vi "Read Order Items.vi"(8 "error in (no error)":errorcluster, 11 "Order in":refnum<class "Order.lvclass">) -> (0 "error out":errorcluster, 2 "Items":refnum<class "Order Item.lvclass">[](array[class]), 3 "Order out":refnum<class "Order.lvclass">)   [LabVIEW 2020, in "Order.lvclass"]
doc: "Simple accessor method to read the items contained in the Order."
uses:
  Order.lvclass
  Order Item/Order Item.lvclass
  Order.lvclass/Order.ctl
  Processes/People/Customers/Customer/Customer.lvclass
  C:/Users/anton/Documents/GitHub/Triarc-Examples/Coffee Shop/Process Job/Job Handler.lvclass
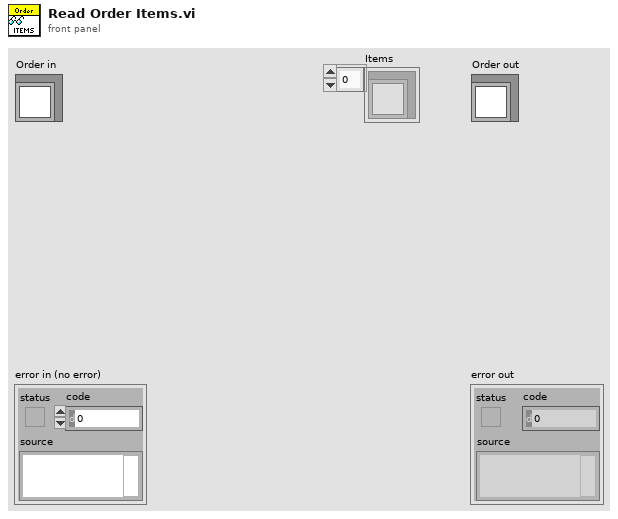
[diagram p1: front panel]
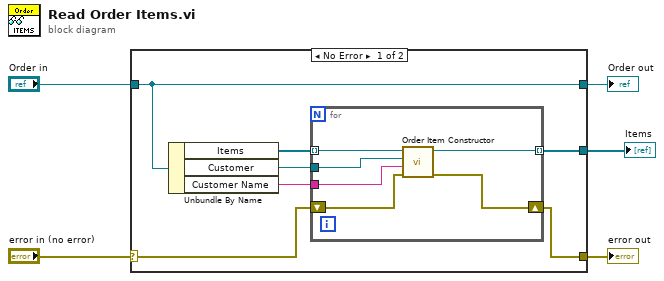
[diagram p0: block diagram]
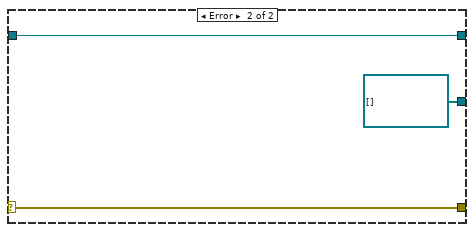
[diagram p2: hidden frame]
diagram:
  n1 = case shown="No Error" "error in (no error)" {
    selector: "error in (no error)" -> [w10 w20]
    tunnel: [w9 w20] -> w4
    tunnel: [w12 w21] -> w2
    tunnel: "Order in" -> [w12 w21]
    tunnel: [w6 refnum<class "Order Item.lvclass">[] []] -> w1
    frame No Error {
      n2 = Unbundle By Name(w12) -> ("Items"=w11:refnum<class "Beverage.lvclass">[], "Customer"=w8:refnum<class "Customer.lvclass">, "Customer Name"=w7:string)
      n3 = for {
        tunnel: w11 -> [w18] mode=indexing
        shift-right: [w16] -> w9
        shift-left: w10 -> [w17]
        tunnel: w8 -> [w15]
        tunnel: w7 -> [w14]
        tunnel: [w13] -> w6 mode=indexing
        n4 = call "Order Item Constructor.vi"("error in (no error)"=w17, "Cust Name"=w14, "Pick Up Order Handler"=w15, "Beverage"=w18) -> ("error out"=w16:errorcluster, "Order Item"=w13:refnum<class "Order Item.lvclass">)  [unwired: 6 in]
      }
    }
    frame Error {
    }
  }
  "error out" <- w4
  "Order out" <- w2
  "Items" <- w1
